vi "Set X-Y ROI.vi"(8 "error in (no error)":errorcluster, 9 "ROI X":cluster{"Index":u32, "Length":u32}, 10 "ROI Y":cluster{"Index":u32, "Length":u32}, 11 "TG Base Graph in":refnum<class "Base Graph.lvclass">) -> (0 "error out":errorcluster, 3 "TG Base Graph out":refnum<class "Base Graph.lvclass">)   [LabVIEW 2023, in "Base Graph.lvclass"]
uses:
  Base Graph.lvclass
  Base Graph.lvclass/Base Graph.ctl
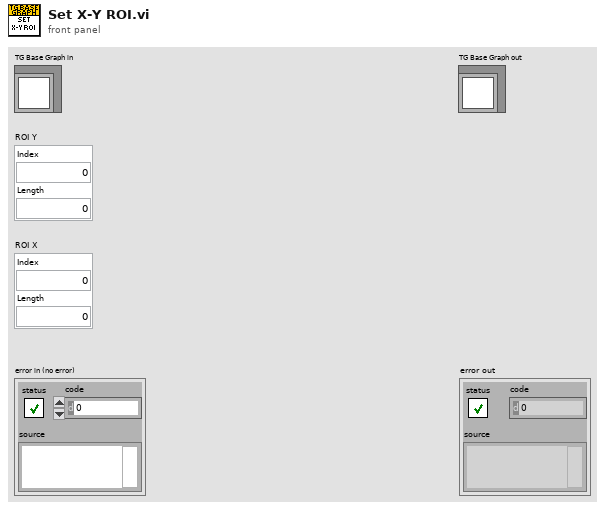
[diagram p1: front panel]
types:
  T1 = cluster{"ROI X":cluster{"Index":u32, "Length":u32}, "ROI Y":cluster{"Index":u32, "Length":u32}}
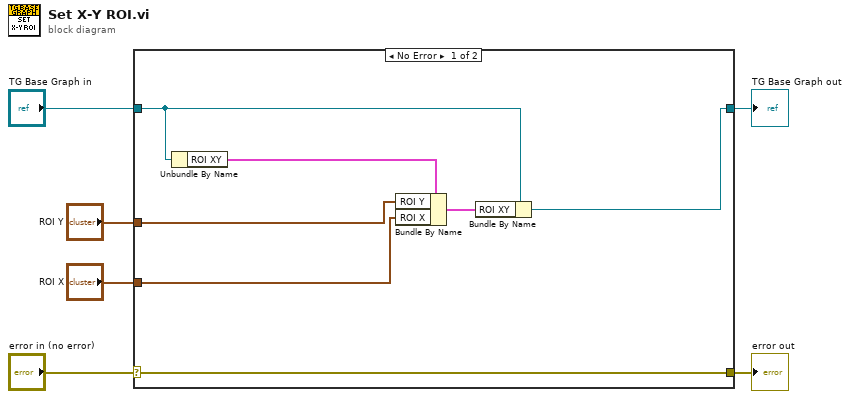
[diagram p0: block diagram]
diagram:
  n1 = case shown="No Error" "error in (no error)" {
    selector: "error in (no error)" -> [w7 w15]
    tunnel: [w7 w15] -> w5
    tunnel: [w9 w14] -> w3
    tunnel: "TG Base Graph in" -> [w10 w14]
    tunnel: "ROI Y" -> [w12 _]
    tunnel: "ROI X" -> [w11 _]
    frame No Error {
      n2 = Unbundle By Name(w10) -> ("ROI XY"=w13:T1)
      n3 = Bundle By Name(cluster=w13, "ROI Y"=w12, "ROI X"=w11) -> (w8:T1)
      n4 = Bundle By Name(cluster=w10, "ROI XY"=w8) -> (w9:refnum<class "Base Graph.lvclass">)
    }
    frame Error {
    }
  }
  "error out" <- w5
  "TG Base Graph out" <- w3
